vi "Hardware Selection.vi"(7 "Command":T1, 8 "error in (no error)":errorcluster) -> (0 "error out":errorcluster, 2 "Module Name":string[](array[string])=["Database", "CAN", "DAQ Hardware", "DAQ IO", "ARINC", "DC Power Supply", "DMM", "Function Generator", "Oscilloscope", "S-Matrix", "Env-Chamber", "CVT", "User Interface"], 3 "Hardware Selection":string[](array[string]))   [LabVIEW 2016, in "User Interface.lvlib"]
uses:
  User Interface.lvlib
  Hardware Selection Command.ctl
  Create Path Command.ctl
  <vilib>/Utility/config.llb/Write Key (String).vi
  <vilib>/Utility/config.llb/Read Key (String).vi
  <vilib>/Utility/config.llb/NI_LVConfig.lvlib
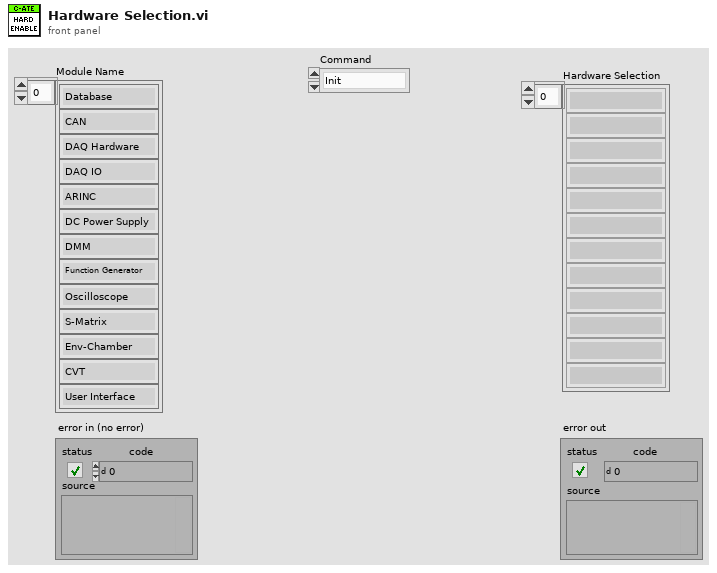
[diagram p1: front panel]
types:
  T1 = typedef "User Interface.lvlib/Hardware Selection Command.ctl" = enum16{"Init", "Read", "Write", "Close"}
  T2 = typedef "User Interface.lvlib/Create Path Command.ctl" = enum16{"Authentication", "Hardware", "Configuration", "Calibration", "Instrument", "Test Description", "Serial Data", "ARINC Data", "CAN Data", "Data", "Report", "Action log", "Error Log"}
  T3 = typedef "NI_LVConfig.lvlib/Config Data RefNum.ctl" = refnum<k1>
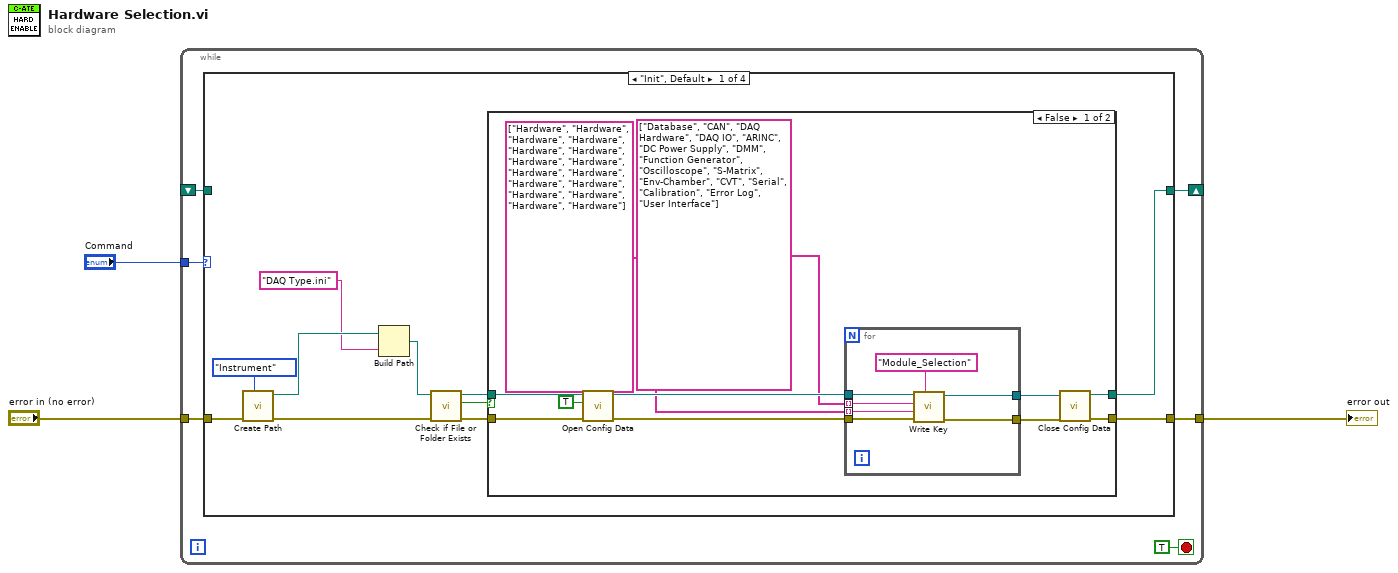
[diagram p0: block diagram]
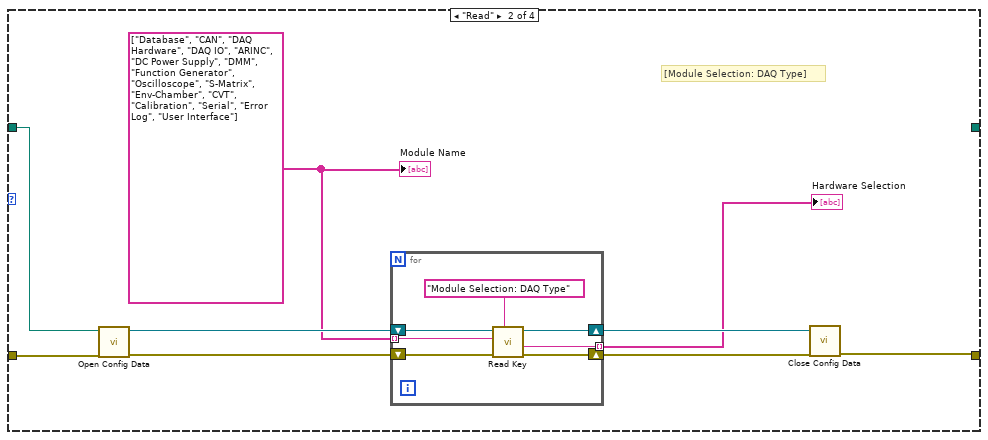
[diagram p3: hidden frame]
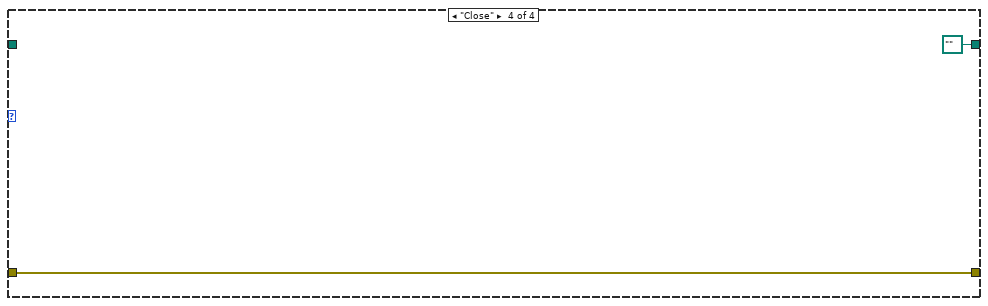
[diagram p5: hidden frame]
diagram:
  n1 = while {
    tunnel: "error in (no error)" -> [w7]
    tunnel: [w6] -> w1
    tunnel: "Command" -> [w8]
    shift-right: [w5] -> _
    shift-left: _ -> [w4]
    stop <- TRUE stop-if-true
    n2 = case shown="\"Init\", Default" w8 {
      tunnel: w7 -> [w19 w49 _ w57]
      tunnel: [w11 w43 _ w57] -> w6
      tunnel: [w10 _ _ path "" ("dup path")] -> w5
      tunnel: w4 -> [_ w48 _ _]
      frame "Init", Default {
        n3 = call "Create Path.vi"("Path Command"=Create_Path_Command."Instrument", "error in (no error)"=w19) -> ("error out"=w15:errorcluster, "created path"=w18:path)  [unwired: 8 in]
        n4 = Build Path(base path=w18, name or relative path="DAQ Type.ini") -> (appended path=w16:path)
        n5 = call <vilib>:"Check if File or Folder Exists.vi"("error in (no error)"=w15, "path"=w16) -> ("error out"=w14:errorcluster, "file or folder exists?"=w13:bool, "dup path"=w12:path)  [unwired: 7 in]
        n6 = case shown="False" w13 {
          tunnel: w14 -> [w30 w40]
          tunnel: w12 -> [w31 w39]
          tunnel: [w26 w40] -> w11
          tunnel: [w23 w39] -> w10
          frame False {
            n7 = call <vilib>:"Open Config Data.vi"("error in (no error)"=w30, "create file if necessary (T)"=TRUE, "configuration file path"=w31) -> ("error out"=w28:errorcluster, "refnum"=w25:T3)  [unwired: 6 in, 1 out]
            n8 = for {
              tunnel: w28 -> [w38]
              tunnel: [w37] -> w27
              tunnel: w25 -> [w36]
              tunnel: [w35] -> w24
              tunnel: string[] ["Database", "CAN", "DAQ Hardware", "DAQ IO", "ARINC", "DC Power Supply", "DMM", "Function Generator", "Oscilloscope", "S-Matrix", "Env-Chamber", "CVT", "Serial", "Calibration", "Error Log", "User Interface"] -> [w33] mode=indexing
              tunnel: string[] ["Hardware", "Hardware", "Hardware", "Hardware", "Hardware", "Hardware", "Hardware", "Hardware", "Hardware", "Hardware", "Hardware", "Hardware", "Hardware", "Hardware", "Hardware", "Hardware"] -> [w32] mode=indexing
              n9 = call-poly <vilib>:"Write Key.vi"("section"="Module_Selection", "error in (no error)"=w38, "value"=w32, "key"=w33, "refnum"=w36) -> ("error out"=w37:errorcluster, "refnum out"=w35:T3)  [unwired: 4 in, 1 out]
            }
            n10 = call <vilib>:"Close Config Data.vi"("error in (no error)"=w27, "refnum"=w24) -> ("error out"=w26:errorcluster, "file path"=w23:path)  [unwired: 8 in]
          }
          frame True {
          }
        }
      }
      frame "Read" {
        w42 = string[] ["Database", "CAN", "DAQ Hardware", "DAQ IO", "ARINC", "DC Power Supply", "DMM", "Function Generator", "Oscilloscope", "S-Matrix", "Env-Chamber", "CVT", "Calibration", "Serial", "Error Log", "User Interface"]
        # "[Module Selection: DAQ Type]"
        n11 = call <vilib>:"Open Config Data.vi"("error in (no error)"=w49, "configuration file path"=w48) -> ("error out"=w46:errorcluster, "refnum"=w47:T3)  [unwired: 7 in, 1 out]
        n12 = for {
          shift-right: [w54] -> w45
          shift-left: w47 -> [w56]
          shift-right: [w53] -> w44
          shift-left: w46 -> [w55]
          tunnel: w42 -> [w51] mode=indexing
          tunnel: [w50] -> w41 mode=indexing
          n13 = call-poly <vilib>:"Read Key.vi"("section"="Module Selection: DAQ Type", "error in (no error)"=w55, "key"=w51, "refnum"=w56) -> ("error out"=w53:errorcluster, "value"=w50:string, "refnum out"=w54:T3)  [unwired: 4 in, 1 out]
        }
        "Hardware Selection" <- w41
        n14 = call <vilib>:"Close Config Data.vi"("error in (no error)"=w44, "refnum"=w45) -> ("error out"=w43:errorcluster)  [unwired: 8 in, 1 out]
        "Module Name" <- w42
      }
      frame "Write" {
      }
      frame "Close" {
      }
    }
  }
  "error out" <- w1
